vi "clLabview_getBlockIdByName.vi"(7 "use compression (off)":bool, 8 "Block Number (0)":u32, 9 "Block Name":string, 10 "vi_lib.lvlib:clLabview.lvclass":refnum<class "clLabview.lvclass">) -> (0 "Block Content":refnum<class "clFileReader.lvclass">, 2 "Name found?":bool)   [LabVIEW 2011, in "vi_lib.lvlib" / "clLabview.lvclass"]
uses:
  clLabview.lvclass
  clFileReader/clFileReader.lvclass
  clLabview.lvclass/clLabview.ctl
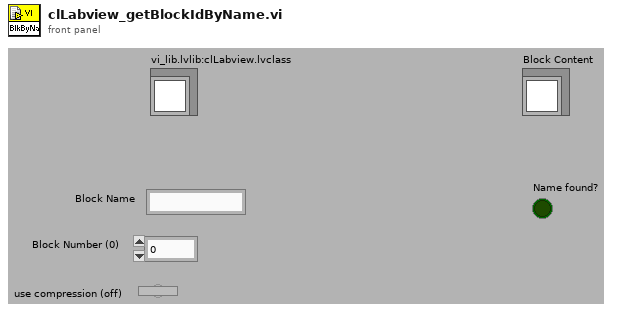
[diagram p1: front panel]
types:
  T1 = cluster{"BlockInfoOffset":u32, "BlockCount":u32, "BlockName":string, "INT2":u32, "INT3":u32, "INT1":u32, "BlockOffset":u32, "INT4":u32, "BlockFileSize":u32}[]
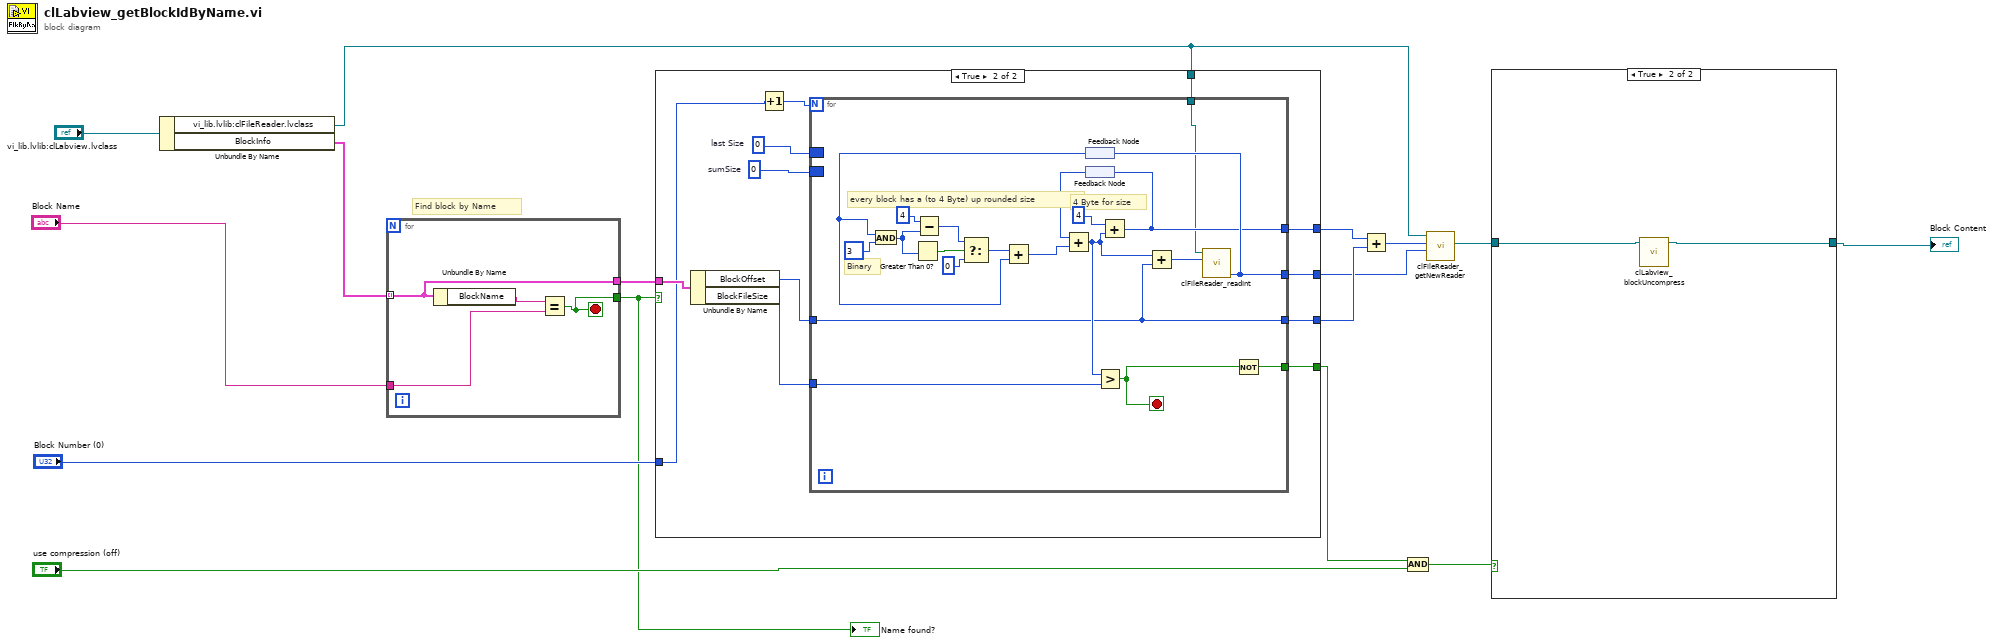
[diagram p0: block diagram]
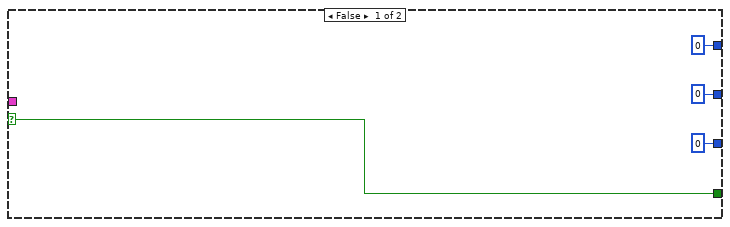
[diagram p3: hidden frame]
diagram:
  # "Find block by Name"
  n1 = Unbundle By Name("vi_lib.lvlib:clLabview.lvclass") -> ("vi_lib.lvlib:clFileReader.lvclass"=w7:refnum<class "clFileReader.lvclass">, "BlockInfo"=w15:T1)
  n2 = for {
    tunnel: w15 -> [w18] mode=indexing
    tunnel: "Block Name" -> [w20]
    tunnel: [w18] -> w13
    tunnel: [w17] -> w1
    stop <- w17 stop-if-true
    n3 = Unbundle By Name(w18) -> ("BlockName"=w19:string)
    n4 = Equal?(x=w19, y=w20) -> (x = y?=w17:bool)
  }
  "Name found?" <- w1
  n5 = case shown="True" w1 {
    selector: w1 -> [w24 _]
    tunnel: w13 -> [_ w36]
    tunnel: "Block Number (0)" -> [_ w25]
    tunnel: [w24 w31] -> w5
    tunnel: [u32 0 w30] -> w11
    tunnel: [u32 0 ("BlockOffset") w29] -> w10
    tunnel: [u32 0 ("OUT Value") w28] -> w9
    tunnel: w7 -> [_ w27]
    frame False {
    }
    frame True {
      w33 = u32 0  # sumSize
      w35 = u32 0  # last Size
      n6 = Unbundle By Name(w36) -> ("BlockOffset"=w34:u32, "BlockFileSize"=w32:u32)
      n7 = Increment(x=w25) -> (x+1=w26:u32)
      n8 = for {
        N: w26 -> [_]
        border: w35 -> [_]
        tunnel: w34 -> [w40]
        border: w33 -> [_]
        tunnel: w32 -> [w43]
        tunnel: [w41] -> w31
        tunnel: [w38] -> w30
        tunnel: [w40] -> w29
        tunnel: [w39] -> w28
        tunnel: w27 -> [w37]
        stop <- w42 stop-if-true
        # "Binary"
        # "4 Byte for size"
        # "every block has a (to 4 Byte) up rounded size"
        n9 = feedback #1() -> (w52:u32)
        n10 = And(x=w52, y=u32 3) -> (x .and. y?=w51:u32)
        n11 = Greater Than 0?(x=w51) -> (x > 0?=w55:bool)
        n12 = Subtract(x=u32 4, y=w51) -> (x-y=w50:u32)
        n13 = Select(t=w50, s=w55, f=u32 0) -> (s? t:f=w53:u32)
        n14 = Add(x=w53, y=w52) -> (x+y=w46:u32)
        n15 = feedback #2() -> (w47:u32)
        n16 = Add(x=w47, y=w46) -> (x+y=w44:u32)
        n17 = Greater?(x=w44, y=w43) -> (0:w42:bool)
        n18 = Add(x=u32 4, y=w44) -> (x+y=w38:u32)
        n19 = feedback-in #2(w38) -> ()
        n20 = Add(x=w44, y=w40) -> (x+y=w48:u32)
        n21 = call "clFileReader_readInt.vi"("offset"=w48, "clFileReader.lvclass IN"=w37) -> ("OUT Value"=w39:u32)  [unwired: 1 in, 8 out]
        n22 = feedback-in #1(w39) -> ()
        n23 = Not(x=w42) -> (.not. x?=w41:bool)
      }
    }
  }
  n24 = Add(x=w11, y=w10) -> (x+y=w8:u32)
  n25 = And(x=w5, y="use compression (off)") -> (x .and. y?=w6:bool)
  n26 = call "clFileReader_getNewReader.vi"("DataLenght"=w9, "HiddenOffset"=w8, "clFileReader.lvclass"=w7) -> ("New clFileReader"=w3:refnum<class "clFileReader.lvclass">)  [unwired: 8 out]
  n27 = case shown="True" w6 {
    tunnel: w3 -> [w57 w59]
    tunnel: [w57 w58] -> w2
    frame False {
    }
    frame True {
      n28 = call "clLabview_blockUncompress.vi"("vi_lib.lvlib:clFileReader.lvclass"=w59) -> ("vi_lib.lvlib:clFileReader.lvclass 2"=w58:refnum<class "clFileReader.lvclass">)  [unwired: 10 out]
    }
  }
  "Block Content" <- w2
